vi "Errors.vi"(2 "Scan Error":refnum<vi>, 3 "IGC100 B Error":refnum<vi>, 5 "6487 Error":refnum<vi>, 6 "ERROR":refnum<vi>, 7 "6485 Error":refnum<vi>, 8 "IGC100 A Error":refnum<vi>, 9 "EG Error":refnum<vi>, 10 "Motor Error":refnum<vi>, 11 "QUIT":refnum<vi>) -> ()   [LabVIEW 2018]
uses:
  <vilib>/Utility/error.llb/DialogType.ctl
panel:
  in  "Select Sub-System":string(combo)
  out "Error Source":string
  out "Error Message":string=" INSTRUCTIONS:\r\rNormal Use:  When using subVIs that incorporate the error in/error out (or error I/O) structure, place this handler where you want to inform the user of an error, typically at the end of the I/O data path, as the last action of the program.  If the error in error? is ERROR, the handler creates a message describing the error and its source.  If the type of dialog = 1 (default), the message is displayed to the user, who can only acknowedge it.  If the type = 2, the user can acknowledge the message or abort execution; aborting a program with active I/O is not recommended.  If the type = 0, no message is displayed; this is used to process the error programmatically, and the error out cluster elements are wired to individual terminals for that reason.  \r\rOther Use:\n\r\nlocal testing.  To test the error code of a subVI or function that does not have the error I/O structure, you can wire its error code and a source string to the local error code and error source inputs.  If error in error? indicates no error and error code is not equal to 0, the local code and source are substituted for the error in values, and error? is set TRUE (ERROR)."
  in  "Clear Error":bool
  out "Error Code":i32 format="%0.0f"
  out "Scan Error":bool
  out "Keithley 6487 Error":bool
  out "Keithley 6485 Error":bool
  out "IGC100 A Error":bool
  out "IGC100 B Error":bool
  out "Motors Error":bool
  out "Staib EG Error":bool
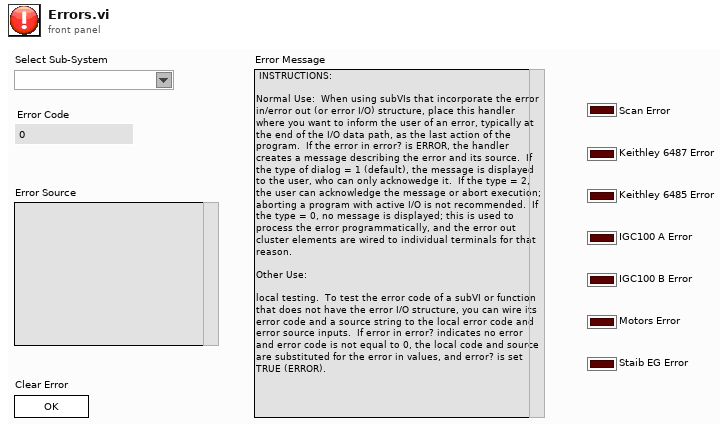
[diagram p1: front panel]
types:
  T1 = typedef "DialogType.ctl" = u16
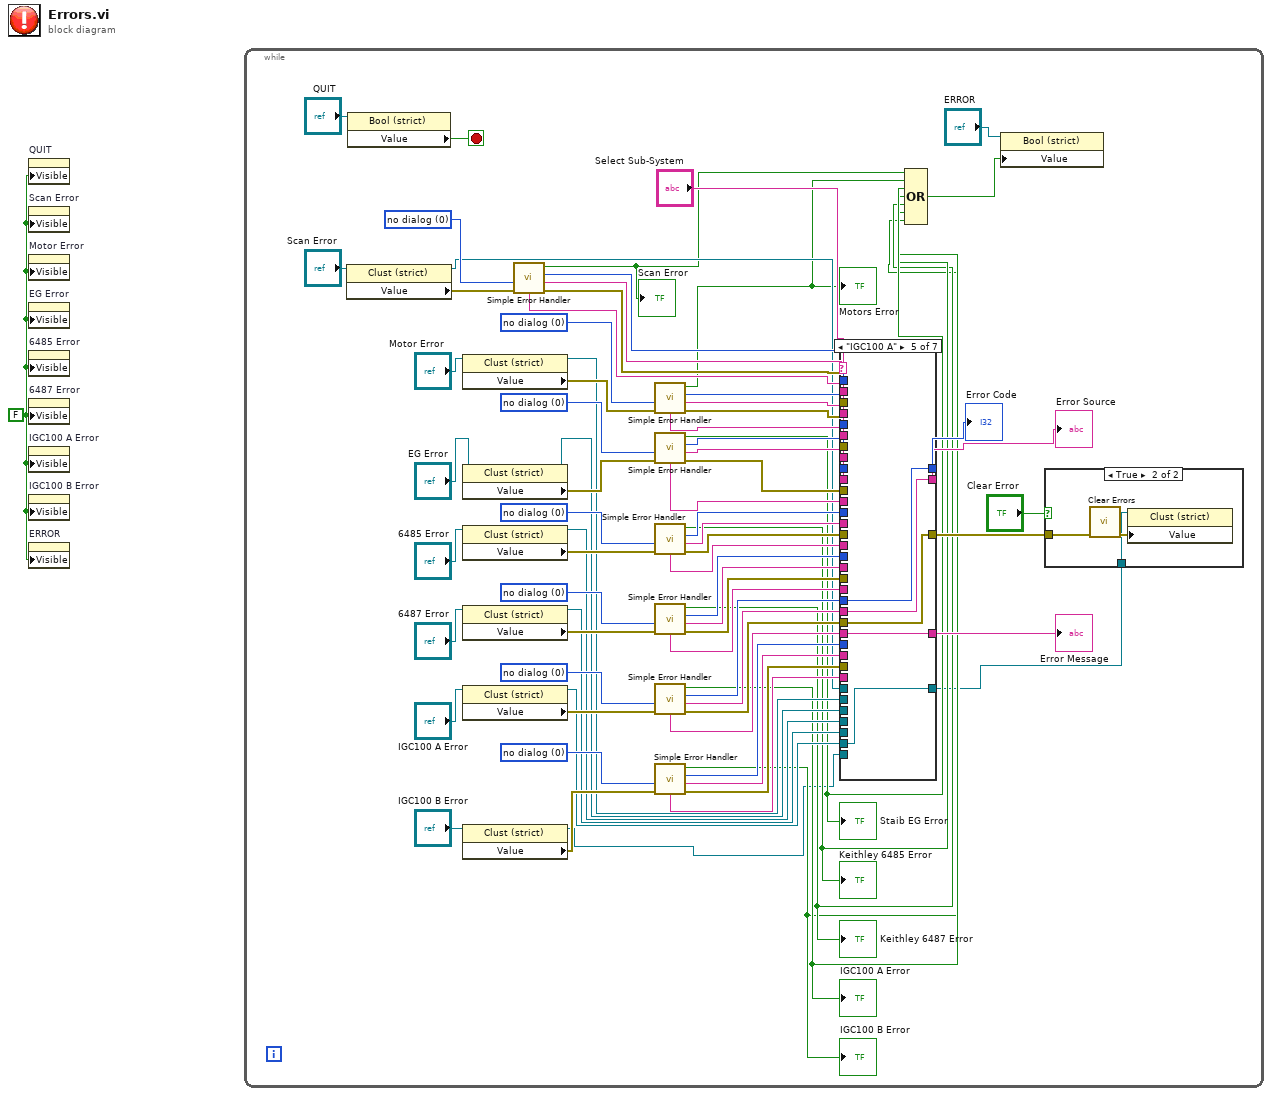
[diagram p0: block diagram]
diagram:
  w1 = FALSE ("Visible")
  n1 = property on="QUIT" class="LVObjRef (strict)"("Visible"=w1) -> ()  [unwired: 2 in, 2 out]
  n2 = property on="Scan Error" class="LVObjRef (strict)"("Visible"=w1) -> ()  [unwired: 2 in, 2 out]
  n3 = property on="Motor Error" class="LVObjRef (strict)"("Visible"=w1) -> ()  [unwired: 2 in, 2 out]
  n4 = property on="EG Error" class="LVObjRef (strict)"("Visible"=w1) -> ()  [unwired: 2 in, 2 out]
  n5 = property on="6485 Error" class="LVObjRef (strict)"("Visible"=w1) -> ()  [unwired: 2 in, 2 out]
  n6 = property on="6487 Error" class="LVObjRef (strict)"("Visible"=w1) -> ()  [unwired: 2 in, 2 out]
  n7 = property on="IGC100 A Error" class="LVObjRef (strict)"("Visible"=w1) -> ()  [unwired: 2 in, 2 out]
  n8 = property on="IGC100 B Error" class="LVObjRef (strict)"("Visible"=w1) -> ()  [unwired: 2 in, 2 out]
  n9 = property on="ERROR" class="LVObjRef (strict)"("Visible"=w1) -> ()  [unwired: 2 in, 2 out]
  n10 = while {
    stop <- w28 stop-if-true
    w55 = T1 0 items=["no dialog", "OK message", "continue or stop message", "OK message + warnings", "continue/stop + warnings"] ("type of dialog (OK msg:1)")
    w70 = T1 0 items=["no dialog", "OK message", "continue or stop message", "OK message + warnings", "continue/stop + warnings"] ("type of dialog (OK msg:1)")
    w69 = T1 0 items=["no dialog", "OK message", "continue or stop message", "OK message + warnings", "continue/stop + warnings"] ("type of dialog (OK msg:1)")
    w68 = T1 0 items=["no dialog", "OK message", "continue or stop message", "OK message + warnings", "continue/stop + warnings"] ("type of dialog (OK msg:1)")
    w67 = T1 0 items=["no dialog", "OK message", "continue or stop message", "OK message + warnings", "continue/stop + warnings"] ("type of dialog (OK msg:1)")
    w66 = T1 0 items=["no dialog", "OK message", "continue or stop message", "OK message + warnings", "continue/stop + warnings"] ("type of dialog (OK msg:1)")
    w59 = T1 0 items=["no dialog", "OK message", "continue or stop message", "OK message + warnings", "continue/stop + warnings"] ("type of dialog (OK msg:1)")
    n11 = property class="Clust (strict)"(reference="Scan Error") -> (reference out=w18:refnum<vi>, "Value"=w72:errorcluster)  [unwired: 1 in, 1 out]
    n12 = property class="Bool (strict)"(reference="QUIT") -> ("Value"=w28:bool)  [unwired: 1 in, 2 out]
    n13 = property class="Clust (strict)"(reference="Motor Error") -> (reference out=w17:refnum<vi>, "Value"=w54:errorcluster)  [unwired: 1 in, 1 out]
    n14 = property class="Clust (strict)"(reference="EG Error") -> (reference out=w13:refnum<vi>, "Value"=w58:errorcluster)  [unwired: 1 in, 1 out]
    n15 = property class="Clust (strict)"(reference="6485 Error") -> (reference out=w16:refnum<vi>, "Value"=w71:errorcluster)  [unwired: 1 in, 1 out]
    n16 = property class="Clust (strict)"(reference="6487 Error") -> (reference out=w15:refnum<vi>, "Value"=w75:errorcluster)  [unwired: 1 in, 1 out]
    n17 = property class="Clust (strict)"(reference="IGC100 A Error") -> (reference out=w14:refnum<vi>, "Value"=w74:errorcluster)  [unwired: 1 in, 1 out]
    n18 = property class="Clust (strict)"(reference="IGC100 B Error") -> (reference out=w3:refnum<vi>, "Value"=w73:errorcluster)  [unwired: 1 in, 1 out]
    n19 = call <vilib>:"Simple Error Handler.vi"("type of dialog (OK msg:1)"=w69, "error in (no error)"=w72) -> ("error?"=w12:bool, "code out"=w50:i32, "source out"=w48:string, "error out"=w19:errorcluster, "message"=w52:string)  [unwired: 3 in]
    "Scan Error" <- w12
    n20 = call <vilib>:"Simple Error Handler.vi"("type of dialog (OK msg:1)"=w55, "error in (no error)"=w54) -> ("error?"=w11:bool, "code out"=w30:i32, "source out"=w31:string, "error out"=w25:errorcluster, "message"=w32:string)  [unwired: 3 in]
    "Motors Error" <- w11
    n21 = call <vilib>:"Simple Error Handler.vi"("type of dialog (OK msg:1)"=w59, "error in (no error)"=w58) -> ("error?"=w10:bool, "code out"=w33:i32, "source out"=w34:string, "error out"=w20:errorcluster, "message"=w35:string)  [unwired: 3 in]
    "Staib EG Error" <- w10
    n22 = call <vilib>:"Simple Error Handler.vi"("type of dialog (OK msg:1)"=w70, "error in (no error)"=w71) -> ("error?"=w9:bool, "code out"=w45:i32, "source out"=w46:string, "error out"=w24:errorcluster, "message"=w47:string)  [unwired: 3 in]
    "Keithley 6485 Error" <- w9
    n23 = call <vilib>:"Simple Error Handler.vi"("type of dialog (OK msg:1)"=w66, "error in (no error)"=w75) -> ("error?"=w8:bool, "code out"=w42:i32, "source out"=w43:string, "error out"=w23:errorcluster, "message"=w44:string)  [unwired: 3 in]
    "Keithley 6487 Error" <- w8
    n24 = call <vilib>:"Simple Error Handler.vi"("type of dialog (OK msg:1)"=w67, "error in (no error)"=w74) -> ("error?"=w7:bool, "code out"=w39:i32, "source out"=w40:string, "error out"=w22:errorcluster, "message"=w41:string)  [unwired: 3 in]
    "IGC100 A Error" <- w7
    n25 = call <vilib>:"Simple Error Handler.vi"("type of dialog (OK msg:1)"=w68, "error in (no error)"=w73) -> ("error?"=w6:bool, "code out"=w36:i32, "source out"=w37:string, "error out"=w21:errorcluster, "message"=w38:string)  [unwired: 3 in]
    "IGC100 B Error" <- w6
    n26 = case shown="\"IGC100 A\"" "Select Sub-System" {
      tunnel: [w83 w88 w93 w98 w103 w108 w113] -> w53
      tunnel: w52 -> [w83 _ _ _ _ _ _]
      tunnel: [w82 w86 w91 w96 w101 w106 w111] -> w51
      tunnel: w50 -> [w82 _ _ _ _ _ _]
      tunnel: [w81 w87 w92 w97 w102 w107 w112] -> w49
      tunnel: w48 -> [w81 _ _ _ _ _ _]
      tunnel: w47 -> [_ _ w93 _ _ _ _]
      tunnel: w46 -> [_ _ w92 _ _ _ _]
      tunnel: w45 -> [_ _ w91 _ _ _ _]
      tunnel: w44 -> [_ _ _ w98 _ _ _]
      tunnel: w43 -> [_ _ _ w97 _ _ _]
      tunnel: w42 -> [_ _ _ w96 _ _ _]
      tunnel: w41 -> [_ _ _ _ w103 _ _]
      tunnel: w40 -> [_ _ _ _ w102 _ _]
      tunnel: w39 -> [_ _ _ _ w101 _ _]
      tunnel: w38 -> [_ _ _ _ _ w108 _]
      tunnel: w37 -> [_ _ _ _ _ w107 _]
      tunnel: w36 -> [_ _ _ _ _ w106 _]
      tunnel: w35 -> [_ _ _ _ _ _ w113]
      tunnel: w34 -> [_ _ _ _ _ _ w112]
      tunnel: w33 -> [_ _ _ _ _ _ w111]
      tunnel: w32 -> [_ w88 _ _ _ _ _]
      tunnel: w31 -> [_ w87 _ _ _ _ _]
      tunnel: w30 -> [_ w86 _ _ _ _ _]
      tunnel: [w80 w85 w90 w95 w100 w105 w110] -> w26
      tunnel: w25 -> [_ w85 _ _ _ _ _]
      tunnel: w24 -> [_ _ w90 _ _ _ _]
      tunnel: w23 -> [_ _ _ w95 _ _ _]
      tunnel: w22 -> [_ _ _ _ w100 _ _]
      tunnel: w21 -> [_ _ _ _ _ w105 _]
      tunnel: w20 -> [_ _ _ _ _ _ w110]
      tunnel: w19 -> [w80 _ _ _ _ _ _]
      tunnel: w18 -> [w79 _ _ _ _ _ _]
      tunnel: w17 -> [_ w84 _ _ _ _ _]
      tunnel: w16 -> [_ _ w89 _ _ _ _]
      tunnel: w15 -> [_ _ _ w94 _ _ _]
      tunnel: w14 -> [_ _ _ _ w99 _ _]
      tunnel: w3 -> [_ _ _ _ _ w104 _]
      tunnel: w13 -> [_ _ _ _ _ _ w109]
      tunnel: [w79 w84 w89 w94 w99 w104 w109] -> w2
      frame "Scan", Default {
      }
      frame "Motors" {
      }
      frame "Keithley 6485" {
      }
      frame "Keithley 6487" {
      }
      frame "IGC100 A" {
      }
      frame "IGC100 B" {
      }
      frame "Staib Electron Gun" {
      }
    }
    "Error Code" <- w51
    "Error Message" <- w53
    "Error Source" <- w49
    n27 = Compound Arithmetic op=OR(w12, w11, w10, w9, w8, w7, w6) -> (w4:bool)
    n28 = property class="Bool (strict)"(reference="ERROR", "Value"=w4) -> ()  [unwired: 1 in, 2 out]
    n29 = case shown="True" "Clear Error" {
      tunnel: w26 -> [_ w78]
      tunnel: w2 -> [_ w76]
      frame False {
      }
      frame True {
        n30 = call <vilib>:"Clear Errors.vi"("error in (no error)"=w78) -> ("error out"=w77:errorcluster)  [unwired: 5 in, 1 out]
        n31 = property class="Clust (strict)"(reference=w76, "Value"=w77) -> ()  [unwired: 1 in, 2 out]
      }
    }
  }
